vi "DataLib.unpack subevent data.vi"(1 "subeventData":T2, 5 "error in (no error)":errorcluster) -> (15 "daqObjects":string[](array[string]), 16 "dataDescriptors":T1[](array[typedef]), 17 "subeventData":string[](array[string]), 19 "error out":errorcluster)   [LabVIEW 2014, in "DataLib.lvlib"]
doc: "This routine can be used to unpack subevent data that is obtained from the routine \"CoreLib.unpack event data\"."
uses:
  DataLib.lvlib
  CS_Core/CSSystem/CoreDefs/CoreDefs.rawDataType.ctl
  CS_Core/BaseProcess/BaseProcess.descriptor string definition.ctl
  CS_Core/BaseProcess/BaseProcess.lvlib
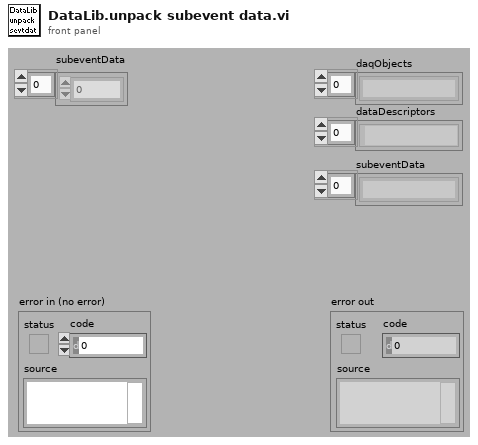
[diagram p1: front panel]
types:
  T1 = typedef "BaseProcess.lvlib/BaseProcess.descriptor string definition.ctl" = string
  T2 = typedef "CoreDefs.rawDataType.ctl" = i8[]
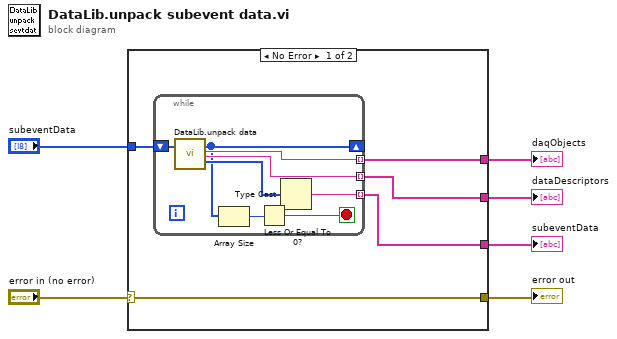
[diagram p0: block diagram]
diagram:
  n1 = case shown="No Error" "error in (no error)" {
    selector: "error in (no error)" -> [w11 w20]
    tunnel: [w7 _] -> w3
    tunnel: "subeventData" -> [w10 _]
    tunnel: [w11 w20] -> w5
    tunnel: [w9 _] -> w1
    tunnel: [w8 _] -> w2
    frame No Error {
      n2 = while {
        tunnel: [w19] -> w7 mode=indexing
        tunnel: [w18] -> w8 mode=indexing
        tunnel: [w12] -> w9 mode=indexing
        shift-right: [w15] -> _
        shift-left: w10 -> [w16]
        stop <- w13 stop-if-true
        n3 = call "DataLib.unpack data.vi"("dataIn"=w16) -> ("remainingData"=w15:T2, "DAQDevice"=w19:string, "Data Descriptor"=w18:T1, "DAQDeviceData"=w17:T2)  [unwired: 14 in, 1 out]
        n4 = Array Size(array=w15) -> (size(s)=w14:i32)
        n5 = Less Or Equal To 0?(x=w14) -> (x <= 0?=w13:bool)
        n6 = Type Cast(x=w17) -> (*(type *) &x=w12:string)  [unwired: 1 in]
      }
    }
    frame Error {
    }
  }
  "error out" <- w5
  "daqObjects" <- w3
  "dataDescriptors" <- w2
  "subeventData" <- w1
